vi "makeManipJump-v02.vi"(0 "which manipulator":T3(ring), 1 "Use Current Position for Start Pos?":bool, 5 "Orig Pos":i32[](array[numeric]), 7 "Which Jumper Position to move to?":T1(ring), 9 "controls array in":refnum<vi>[](array[refnum]), 11 "error in":errorcluster, 12 "common cluster":T2) -> (4 "currentPos":i32[](array[numeric]), 10 "control array out":refnum<vi>[](array[refnum]), 15 "error out":errorcluster)   [LabVIEW 2019]
uses:
  multipatch/controls/multipatch_common_controls_v4.ctl
  machine_vision/controls/transform_cluster_actuator.ctl
  machine_vision/coordinate model vis/transform_properties_actuators.ctl
  pipette cleaning/pressure box/cleaning_soft/controls/actuator_cluster.ctl
  pipette cleaning/pressure box/cleaning_soft/controls/actuator_type.ctl
  pipette cleaning/pressure box/cleaning_soft/controls/pressure_box_control.ctl
  pipette cleaning/pressure box/cleaning_soft/controls/pressure_box_type.ctl
  controls/NH_method.ctl
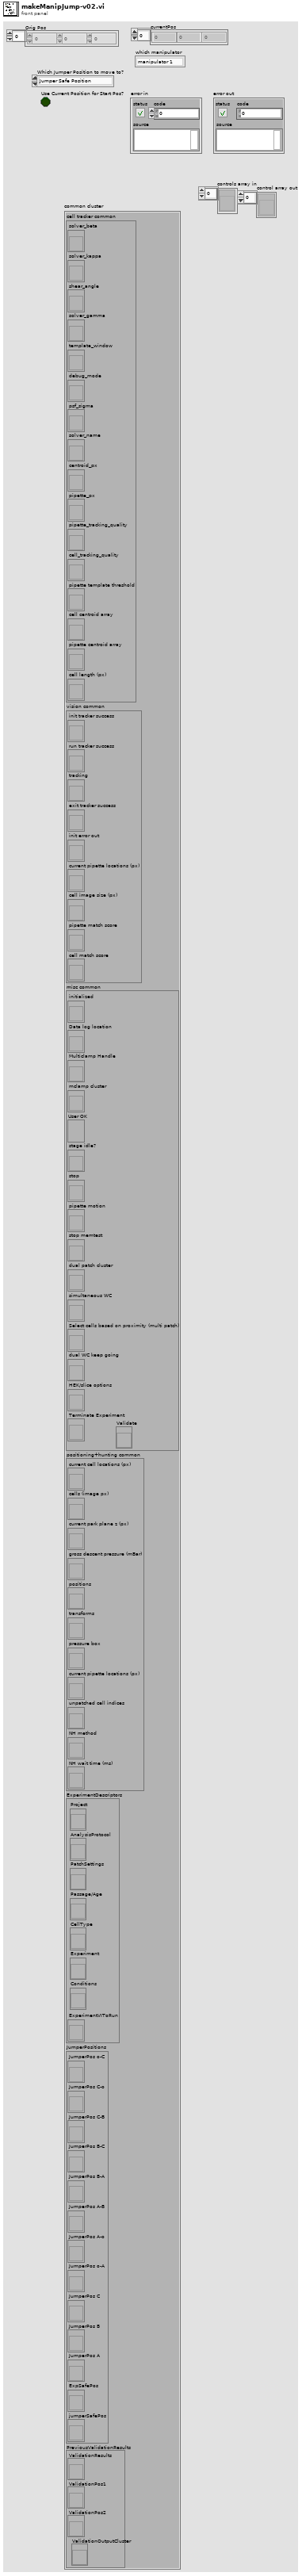
[diagram p1: front panel]
types:
  T1 = enum16{"Jumper Safe Position", "Experiment Safe Position", "Jumper Position A", "Jumper Position B", "Jumper Position C", "Jumper Position o-A", "Jumper Position A-o", "Jumper Position A-B", "Jumper Position B-A", "Jumper Position B-C", "Jumper Position C-B", "Jumper Position C-o", "Jumper Position o-C"}
  T2 = typedef "multipatch_common_controls_v4.ctl" = cluster{"cell tracker common":cluster{"solver_beta":refnum<vi>, "solver_kappa":refnum<vi>, "shear_angle":refnum<vi>, "solver_gamma":refnum<vi>, "template_window":refnum<vi>, "debug_mode":refnum<vi>, "psf_sigma":refnum<vi>, "solver_name":refnum<vi>, "centroid_px":refnum<vi>, "pipette_px":refnum<vi>, "pipette_tracking_quality":refnum<vi>, "cell_tracking_quality":refnum<vi>, "pipette template threshold":refnum<vi>, "cell centroid array":refnum<vi>, "pipette centroid array":refnum<vi>, "cell length (px)":refnum<vi>}, "vision common":cluster{"init tracker success":refnum<vi>, "run tracker success":refnum<vi>, "tracking":refnum<vi>, "exit tracker success":refnum<vi>, "init error out":refnum<vi>, "current pipette locations (px)":refnum<vi>, "cell image size (px)":refnum<vi>, "pipette match score":refnum<vi>, "cell match score":refnum<vi>}, "misc common":cluster{"initialized":refnum<vi>, "Data log location":refnum<vi>, "Multiclamp Handle":refnum<vi>, "mclamp cluster":refnum<vi>, "User OK":refnum<vi>, "stage idle?":refnum<vi>, "stop":refnum<vi>, "pipette motion":refnum<vi>, "stop memtest":refnum<vi>, "dual patch cluster":refnum<vi>, "simultaneous WC":refnum<vi>, "Select cells based on proximity (multi patch)":refnum<vi>, "dual WC keep going":refnum<vi>, "HEK/slice options":refnum<vi>, "Terminate Experiment":refnum<vi>, "Validate":refnum<vi>}, "positioning+hunting common":cluster{"current cell locations (px)":refnum<vi>, "cells (image px)":refnum<vi>, "current park plane z (px)":refnum<vi>, "gross descent pressure (mBar)":refnum<vi>, "positions":refnum<vi>, "transforms":refnum<vi>, "pressure box":refnum<vi>, "current pipette locations (px)":refnum<vi>, "unpatched cell indices":refnum<vi>, "NH method":refnum<vi>, "NH wait time (ms)":refnum<vi>}, "ExperimentDescriptors":cluster{"Project":refnum<vi>, "AnalysisProtocol":refnum<vi>, "PatchSettings":refnum<vi>, "Passage/Age":refnum<vi>, "CellType":refnum<vi>, "Experiment":refnum<vi>, "Conditions":refnum<vi>, "ExperimentVIToRun":refnum<vi>}, "JumperPositions":cluster{"JumperPos o-C":refnum<vi>, "JumperPos C-o":refnum<vi>, "JumperPos C-B":refnum<vi>, "JumperPos B-C":refnum<vi>, "JumperPos B-A":refnum<vi>, "JumperPos A-B":refnum<vi>, "JumperPos A-o":refnum<vi>, "JumperPos o-A":refnum<vi>, "JumperPos C":refnum<vi>, "JumperPos B":refnum<vi>, "JumperPos A":refnum<vi>, "ExpSafePos":refnum<vi>, "jumperSafePos":refnum<vi>}, "PreviousValidationResults":cluster{"ValidationResults":refnum<vi>, "ValidationPos1":refnum<vi>, "ValidationPos2":refnum<vi>, "ValidationOutputCluster":refnum<vi>}}
  T3 = enum16{"manipulator 1", "manipulator 2", "manipulator 3", "manipulator 4"}
  T4 = cluster{"JumperPos o-C":refnum<vi>, "JumperPos C-o":refnum<vi>, "JumperPos C-B":refnum<vi>, "JumperPos B-C":refnum<vi>, "JumperPos B-A":refnum<vi>, "JumperPos A-B":refnum<vi>, "JumperPos A-o":refnum<vi>, "JumperPos o-A":refnum<vi>, "JumperPos C":refnum<vi>, "JumperPos B":refnum<vi>, "JumperPos A":refnum<vi>, "ExpSafePos":refnum<vi>, "jumperSafePos":refnum<vi>}
  T5 = typedef "pressure_box_control.ctl" = cluster{"Pressure box COM":refnum<visa-resource-name>, "pressure box type":T6, "High pos pressure (mBar)":dbl, "Low pos pressure (mBar)":dbl, "Vacuum pressure (mBar)":dbl, "calibration":enum16{"PA_vacPump", "PA_venturi", "Neuromatics", "ilyaRig", "mightenRig"}}
  T6 = typedef "pressure_box_type.ctl" = enum16{"Neuromatics", "ProportionAir", "Demo box", "N-ProportionAir"}
  T7 = cluster{"current stage pos (steps)":refnum<vi>, "current manip 1 pos (steps)":refnum<vi>, "current manip 2 pos (steps)":refnum<vi>, "current manip 3 pos (steps)":refnum<vi>, "current manip 4 pos (steps)":refnum<vi>}
  T8 = typedef "transform_cluster_actuator.ctl" = cluster{"s":refnum<vi>, "manip 1":refnum<vi>, "manip 2":refnum<vi>, "manip 3":refnum<vi>, "manip 4":refnum<vi>}
  T9 = typedef "scope_motion.ctl" = enum16{"superSlow", "fast", "slow", "find slice speed", "slow_dualPatch"}
  T10 = typedef "transform_properties_actuators.ctl" = cluster{"theta (deg)":dbl, "X sc factor (px/step)":dbl, "Y sc factor (px/step)":dbl, "zero loc (x,y,z)":dbl[], "flip y?":bool, "flip x?":bool, "gamma (deg)":dbl, "flip z?":bool, "Z sc factor (px/step)":dbl, "actuator":T11, "safe space (steps)":i32[]}
  T11 = typedef "actuator_cluster.ctl" = cluster{"Actuator COM":refnum<visa-resource-name>, "Actuator type":T12}
  T12 = typedef "actuator_type.ctl" = enum16{"Scientifica", "Sutter", "Demo", "Off"}
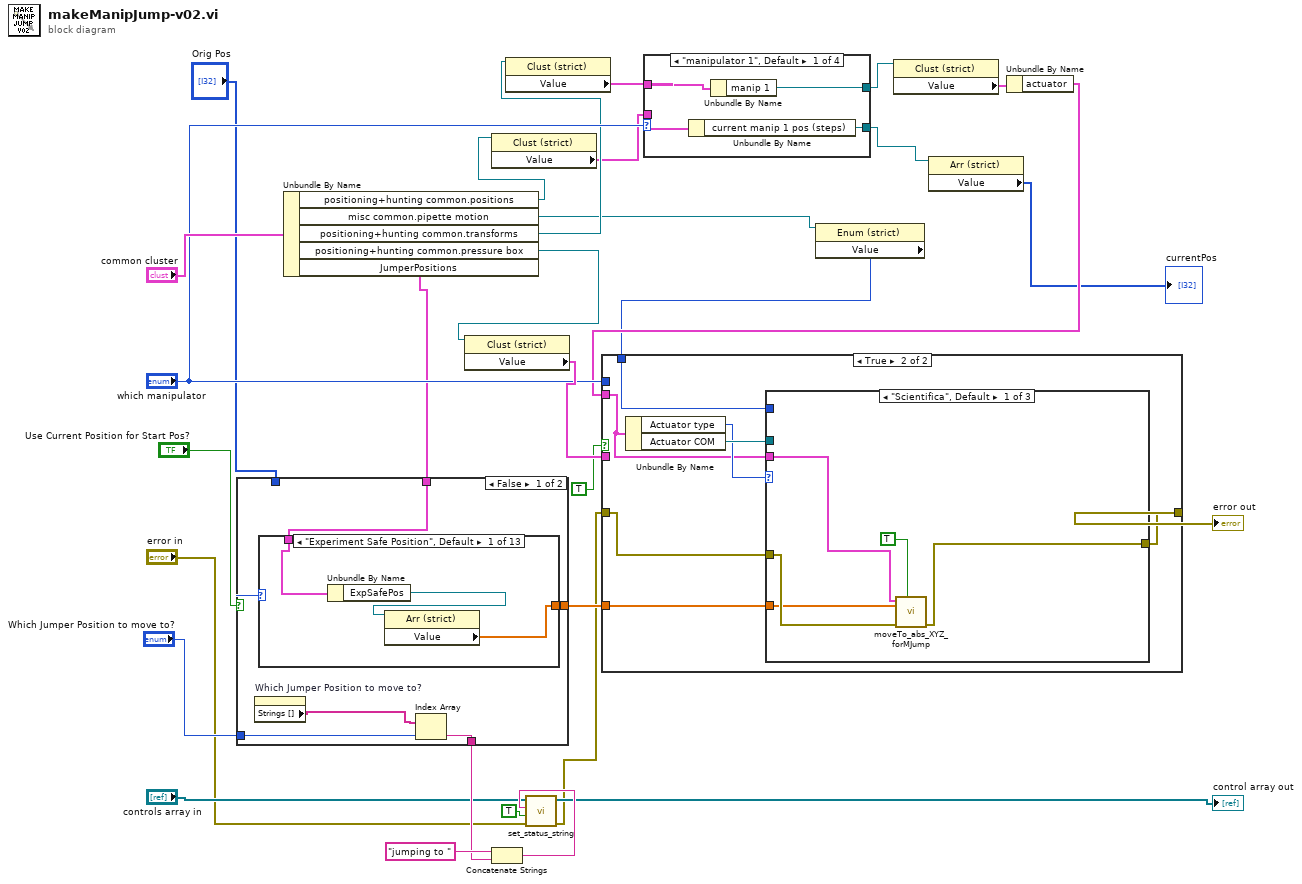
[diagram p0: block diagram]
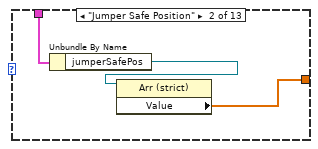
[diagram p2: hidden frame]
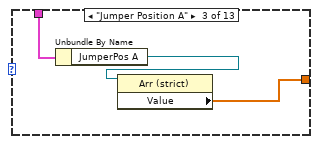
[diagram p3: hidden frame]
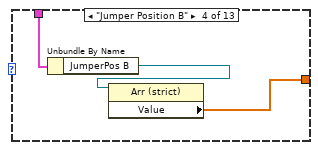
[diagram p4: hidden frame]
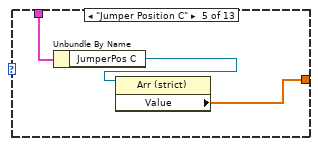
[diagram p5: hidden frame]
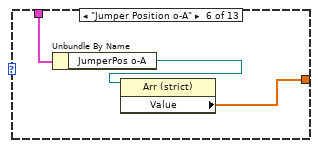
[diagram p6: hidden frame]
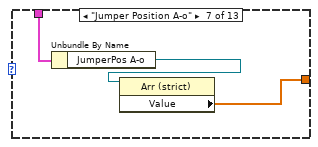
[diagram p7: hidden frame]
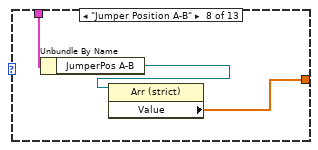
[diagram p8: hidden frame]
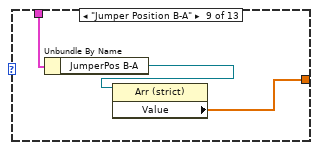
[diagram p9: hidden frame]
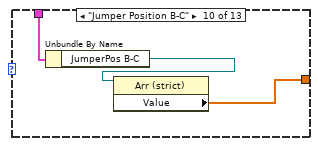
[diagram p10: hidden frame]
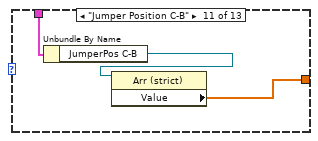
[diagram p11: hidden frame]
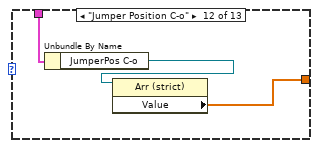
[diagram p12: hidden frame]
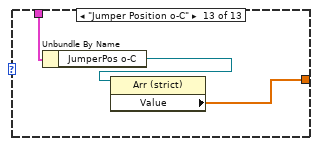
[diagram p13: hidden frame]
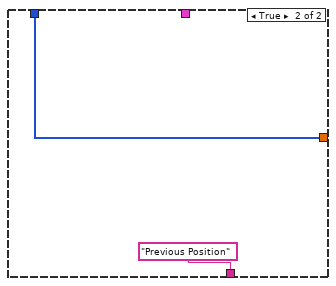
[diagram p14: hidden frame]
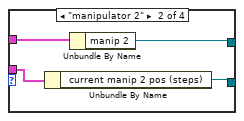
[diagram p15: hidden frame]
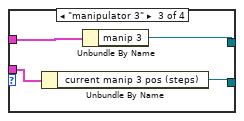
[diagram p16: hidden frame]
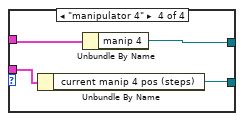
[diagram p17: hidden frame]
diagram:
  n1 = Unbundle By Name("common cluster") -> ("positioning+hunting common.positions"=w15:refnum<vi>, "misc common.pipette motion"=w20:refnum<vi>, "positioning+hunting common.transforms"=w21:refnum<vi>, "positioning+hunting common.pressure box"=w29:refnum<vi>, "JumperPositions"=w14:T4)
  n2 = case shown="False" "Use Current Position for Start Pos?" {
    tunnel: [w35 w76] -> w16
    tunnel: w14 -> [w34 _]
    tunnel: [w33 "Previous Position"] -> w10
    tunnel: "Which Jumper Position to move to?" -> [w32 _]
    tunnel: "Orig Pos" -> [_ w76]
    frame False {
      n3 = property on="Which Jumper Position to move to?" class="Enum (strict)"() -> ("Strings []"=w31:string[])  [unwired: 2 in, 2 out]
      n4 = case shown="\"Experiment Safe Position\", Default" w32 {
        tunnel: [w36 w39 w42 w45 w49 w52 w55 w58 w61 w64 w67 w70 w73] -> w35
        tunnel: w34 -> [w38 w40 w43 w46 w48 w51 w54 w57 w60 w63 w66 w69 w72]
        frame "Experiment Safe Position", Default {
          n5 = Unbundle By Name(w38) -> ("ExpSafePos"=w37:refnum<vi>)
          n6 = property class="Arr (strict)"(reference=w37) -> ("Value"=w36:dbl[])  [unwired: 1 in, 2 out]
        }
        frame "Jumper Safe Position" {
          n7 = Unbundle By Name(w40) -> ("jumperSafePos"=w41:refnum<vi>)
          n8 = property class="Arr (strict)"(reference=w41) -> ("Value"=w39:dbl[])  [unwired: 1 in, 2 out]
        }
        frame "Jumper Position A" {
          n9 = Unbundle By Name(w43) -> ("JumperPos A"=w44:refnum<vi>)
          n10 = property class="Arr (strict)"(reference=w44) -> ("Value"=w42:dbl[])  [unwired: 1 in, 2 out]
        }
        frame "Jumper Position B" {
          n11 = Unbundle By Name(w46) -> ("JumperPos B"=w47:refnum<vi>)
          n12 = property class="Arr (strict)"(reference=w47) -> ("Value"=w45:dbl[])  [unwired: 1 in, 2 out]
        }
        frame "Jumper Position C" {
          n13 = Unbundle By Name(w48) -> ("JumperPos C"=w50:refnum<vi>)
          n14 = property class="Arr (strict)"(reference=w50) -> ("Value"=w49:dbl[])  [unwired: 1 in, 2 out]
        }
        frame "Jumper Position o-A" {
          n15 = Unbundle By Name(w51) -> ("JumperPos o-A"=w53:refnum<vi>)
          n16 = property class="Arr (strict)"(reference=w53) -> ("Value"=w52:dbl[])  [unwired: 1 in, 2 out]
        }
        frame "Jumper Position A-o" {
          n17 = Unbundle By Name(w54) -> ("JumperPos A-o"=w56:refnum<vi>)
          n18 = property class="Arr (strict)"(reference=w56) -> ("Value"=w55:dbl[])  [unwired: 1 in, 2 out]
        }
        frame "Jumper Position A-B" {
          n19 = Unbundle By Name(w57) -> ("JumperPos A-B"=w59:refnum<vi>)
          n20 = property class="Arr (strict)"(reference=w59) -> ("Value"=w58:dbl[])  [unwired: 1 in, 2 out]
        }
        frame "Jumper Position B-A" {
          n21 = Unbundle By Name(w60) -> ("JumperPos B-A"=w62:refnum<vi>)
          n22 = property class="Arr (strict)"(reference=w62) -> ("Value"=w61:dbl[])  [unwired: 1 in, 2 out]
        }
        frame "Jumper Position B-C" {
          n23 = Unbundle By Name(w63) -> ("JumperPos B-C"=w65:refnum<vi>)
          n24 = property class="Arr (strict)"(reference=w65) -> ("Value"=w64:dbl[])  [unwired: 1 in, 2 out]
        }
        frame "Jumper Position C-B" {
          n25 = Unbundle By Name(w66) -> ("JumperPos C-B"=w68:refnum<vi>)
          n26 = property class="Arr (strict)"(reference=w68) -> ("Value"=w67:dbl[])  [unwired: 1 in, 2 out]
        }
        frame "Jumper Position C-o" {
          n27 = Unbundle By Name(w69) -> ("JumperPos C-o"=w71:refnum<vi>)
          n28 = property class="Arr (strict)"(reference=w71) -> ("Value"=w70:dbl[])  [unwired: 1 in, 2 out]
        }
        frame "Jumper Position o-C" {
          n29 = Unbundle By Name(w72) -> ("JumperPos o-C"=w74:refnum<vi>)
          n30 = property class="Arr (strict)"(reference=w74) -> ("Value"=w73:dbl[])  [unwired: 1 in, 2 out]
        }
      }
      n31 = Index Array(array=w31, index=w32) -> (element=w33:string)
    }
    frame True {
    }
  }
  n32 = property class="Clust (strict)"(reference=w29) -> ("Value"=w27:T5)  [unwired: 1 in, 2 out]
  n33 = property class="Clust (strict)"(reference=w15) -> ("Value"=w18:T7)  [unwired: 1 in, 2 out]
  n34 = Concatenate Strings("jumping to " ("string"), w10) -> (w12:string)
  n35 = property class="Clust (strict)"(reference=w21) -> ("Value"=w26:T8)  [unwired: 1 in, 2 out]
  n36 = call "set_status_string.vi"("error in"="error in", "new line?"=TRUE, "status string in"=w12, "controls array"="controls array in") -> ("error out"=w5:errorcluster, "controls array out"=→"control array out":refnum<vi>[])  [unwired: 6 in]
  n37 = case shown="\"manipulator 1\", Default" "which manipulator" {
    tunnel: w26 -> [w80 w84 w88 w92]
    tunnel: [w79 w83 w87 w91] -> w24
    tunnel: w18 -> [w78 w82 w86 w90]
    tunnel: [w77 w81 w85 w89] -> w3
    frame "manipulator 1", Default {
      n38 = Unbundle By Name(w78) -> ("current manip 1 pos (steps)"=w77:refnum<vi>)
      n39 = Unbundle By Name(w80) -> ("manip 1"=w79:refnum<vi>)
    }
    frame "manipulator 2" {
      n40 = Unbundle By Name(w82) -> ("current manip 2 pos (steps)"=w81:refnum<vi>)
      n41 = Unbundle By Name(w84) -> ("manip 2"=w83:refnum<vi>)
    }
    frame "manipulator 3" {
      n42 = Unbundle By Name(w86) -> ("current manip 3 pos (steps)"=w85:refnum<vi>)
      n43 = Unbundle By Name(w88) -> ("manip 3"=w87:refnum<vi>)
    }
    frame "manipulator 4" {
      n44 = Unbundle By Name(w90) -> ("current manip 4 pos (steps)"=w89:refnum<vi>)
      n45 = Unbundle By Name(w92) -> ("manip 4"=w91:refnum<vi>)
    }
  }
  n46 = property class="Enum (strict)"(reference=w20) -> ("Value"=w19:T9)  [unwired: 1 in, 2 out]
  n47 = property class="Clust (strict)"(reference=w24) -> ("Value"=w23:T10)  [unwired: 1 in, 2 out]
  n48 = property class="Arr (strict)"(reference=w3) -> ("Value"=→"currentPos":i32[])  [unwired: 1 in, 2 out]
  n49 = Unbundle By Name(w23) -> ("actuator"=w22:T11)
  n50 = case shown="True" TRUE {
    tunnel: w5 -> [w93 w98]
    tunnel: [w93 w97] -> w28
    tunnel: "which manipulator" -> [_ _]
    tunnel: w27 -> [_ _]
    tunnel: w22 -> [_ w95]
    tunnel: w19 -> [_ w96]
    tunnel: w16 -> [_ w94]
    frame False {
    }
    frame True {
      n51 = Unbundle By Name(w95) -> ("Actuator type"=w99:T12, "Actuator COM"=w100:refnum<visa-resource-name>)
      n52 = case shown="\"Scientifica\", Default" w99 {
        tunnel: w100 -> [_ _ _]
        tunnel: [w101 w106 w107] -> w97
        tunnel: w96 -> [_ _ _]
        tunnel: w95 -> [w105 _ _]
        tunnel: w98 -> [w104 w106 w107]
        tunnel: w94 -> [w103 _ _]
        frame "Scientifica", Default {
          n53 = call "moveTo_abs_XYZ_forMJump.vi"("blocking?"=TRUE, "error in"=w104, "XYZ location (steps)"=w103, "Actuator cluster in"=w105) -> ("error out"=w101:errorcluster)  [unwired: 6 in, 1 out]
        }
        frame "Sutter" {
        }
        frame "Demo" {
        }
      }
    }
  }
  "error out" <- w28
